vi "AsynchronousAPI_TEMPLATE.vi"(8 "error in (no error)":errorcluster, 10 "myData":string, 11 "SMO.jsonRPC":refnum<class "SMO.jsonRPC.lvclass">) -> (0 "error out":errorcluster, 1 "id":i32, 3 "SMO.jsonRPC out":refnum<class "SMO.jsonRPC.lvclass">)   [LabVIEW 2013, in "SMO.jsonRPC.lvclass"]
doc: "---------------------------------------------------------------\nJKI State Machine Objects™\nhttp://jki.net/state-machine-objects/\nCopyright (C) 2005-2015, JKI <info@jki.net>\nALL RIGHTS RESERVEDJKI State Machine Objects (SMO) 1.0.0.5\nJKI - JKI\nCopyright (c) 2016, JKI"
uses:
  SMO.jsonRPC.lvclass
  Typedefs/Request--Cluster.ctl
  <vilib>/JKI/JKI JSON RPC Specification/Request/Request.lvclass
  <vilib>/JKI/JKI JSON RPC Specification/Response/Response.lvclass
panel:
  # "For instructions on how to use the JKI State Machine Objects, examples and video tutorials, visit:\nhttp://jki.net/state-machine-objects/\n\nJKI State Machine Objects™\nhttp://jki.net/state-machine-objects/\nCopyright (C) 2005-2015, JKI <info@jki.net>\nALL RIGHTS RESERVED"
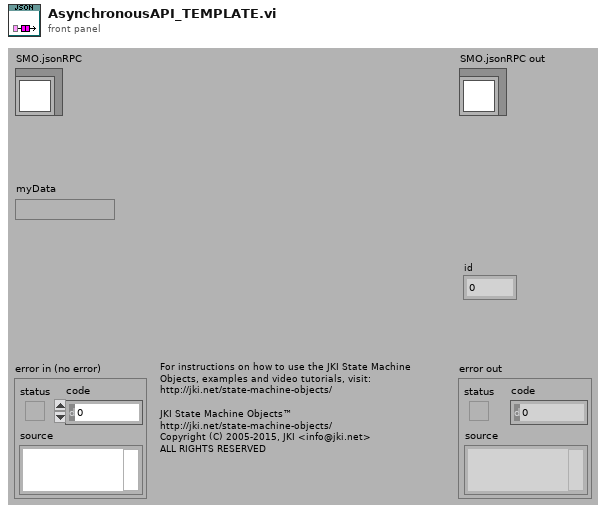
[diagram p1: front panel]
types:
  T1 = typedef "SMO.jsonRPC.lvclass/Request--Cluster.ctl" = cluster{"Request":refnum<class "Request.lvclass">, "reply queue":refnum<queue>, "Async?":bool}
  T2 = typedef "SMO.jsonRPC.lvclass/PrivateEvents--Cluster.ctl" = cluster{"Incoming Request":refnum<user-event>}
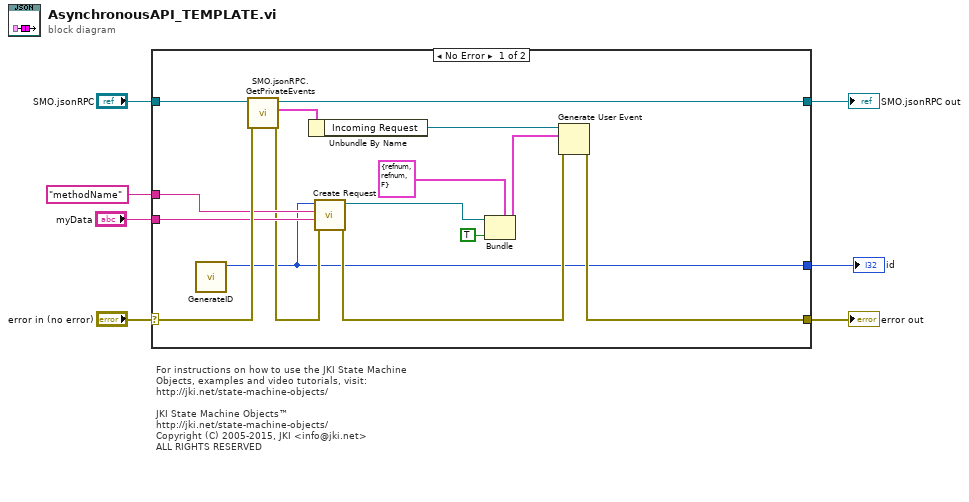
[diagram p0: block diagram]
diagram:
  # "For instructions on how to use the JKI State Machine Objects, examples and video tutorials, visit:\nhttp://jki.net/state-machine-objects/\n\nJKI State Machine Objects™\nhttp://jki.net/state-machine-objects/\nCopyright (C) 2005-2015, JKI <info@jki.net>\nALL RIGHTS RESERVED"
  n1 = case shown="No Error" "error in (no error)" {
    selector: "error in (no error)" -> [w22 w23]
    tunnel: "SMO.jsonRPC" -> [w20 w24]
    tunnel: [w14 w23] -> w6
    tunnel: [w21 w24] -> w5
    tunnel: "myData" -> [w11 _]
    tunnel: "methodName" ("Method") -> [w12 _]
    tunnel: [w8 _] -> w1
    frame No Error {
      n2 = call "GenerateID.vi"() -> ("id"=w8:i32)  [unwired: 11 in]
      n3 = call "SMO.jsonRPC.GetPrivateEvents.vi"("error in (no error)"=w22, "SMO.jsonRPC"=w20) -> ("error out"=w10:errorcluster, "Private Events"=w18:T2, "SMO.jsonRPC out"=w21:refnum<class "SMO.jsonRPC.lvclass">)  [unwired: 7 in]
      n4 = Unbundle By Name(w18) -> ("Incoming Request"=w19:refnum<user-event>)
      n5 = call <vilib>:"Create Request.vi"("error in (no error)"=w10, "Parameters"=w11, "Method"=w12, "id (-1: notification)"=w8) -> ("error out"=w9:errorcluster, "Request"=w13:refnum<class "Request.lvclass">)  [unwired: 5 in, 1 out]
      n6 = Bundle(cluster=T1 {"Request"=refnum, "reply queue"=refnum, "Async?"=FALSE} ("event data"), "Request"=w13, "Async?"=TRUE) -> (w16:T1)  [unwired: 1 in]
      n7 = Generate User Event(user event=w19, event data cluster=w16, error in=w9) -> (error out=w14:errorcluster)  [unwired: 1 in, 1 out]
    }
    frame Error {
    }
  }
  "error out" <- w6
  "SMO.jsonRPC out" <- w5
  "id" <- w1
